vi "BRig_RT__Case_Exp__recordAnalogInput__PortC__fifo__1value__v2.vi"(2 "input_iOccurence":u16, 3 "resetOccurrence":bool, 4 "input_dataCurrent":u16[](array[numeric]), 5 "input_AnaIn_array":i16[][](array[numeric]), 6 "input_iState_start":T1, 7 "rt fifo":refnum<k33>, 8 "input_iState_end":T1, 9 "input_fifo_error":errorcluster) -> (11 "output_fifo_error":errorcluster, 13 "rt fifo out":refnum<k33>, 16 "output_iOccurrence":u16)   [LabVIEW 2014]
uses:
  myRIO_BRig_RT__Case_Exp_stateList.ctl
panel:
  out "anyTimeout":bool
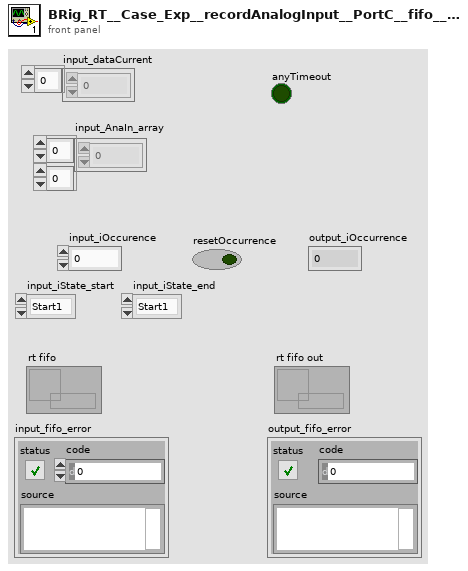
[diagram p1: front panel]
types:
  T1 = typedef "myRIO_BRig_RT__Case_Exp_stateList.ctl" = enum16{"Start1", "Start2", "Start3", "saveSettings1", "saveSettings2", "saveSettings3", "saveSettings4", "saveSettings_LC_ENL_l1", "saveSettings_LC_ENL_l2", "saveSettings_LC_Cue_l1", "saveSettings_LC_Cue_l2", "saveSettings6_LC_l1_Other", "SaveSettings6_LC_l2_Other", "setSettings_Audio", "setSettings_Laser", "initBlock_pre", "initBlock", "initBlock2", "initBlock_post", "initTrial_pre", "initTrial", "initTrial2", "initTrial3", "initTrial4", "initTrial_LC_ENL1", "initTrial_LC_Cue1", "initTrial_LC_Cue1_2", "initTrial_LC_Sel", "initTrial_post", "ENL1_pre", "ENL1", "ENL1_post", "ENL1Penalty_pre", "ENL1Penalty", "ENL2_pre", "ENL2", "ENL2Penalty_pre", "ENL2Penalty", "Cue1_pre", "Cue1", "Cue1_post", "Cue1Penalty_pre", "Cue1Penalty", "Cue2_pre", "Cue2", "Cue2Penalty_pre", "Cue2Penalty", "Selection_pre", "Selection", "Select_post", "SelectReward_pre", "SelectReward", "SelectRewardPost_pre", "SelectRewardPost", "SelectWrong_pre", "SelectWrong", "SelectWrong_post", "SelectTimeout_pre", "SelectTimeout", "SelectTimeout_post", "endTrial_pre", "endTrial1", "endTrial2", "endTrial3", "endTrial_post", "endBlock_pre", "endBlock", "endBlock_post", "endExp", "commConnect", "commUpload_pre", "commUpload_dataBlock", "commUpload_dataCurrent", "commUpload_dataExp", "commUpload_dataLC", "commUpload_dataTrial", "commUpload_post", "saveData_pre", "saveData_dataBlock", "saveData_dataCurrent", "saveData_dataExp", "saveData_dataLC", "saveData_dataTrial", "saveData_post", "empty_endBlock1", "empty_endBlock2", "empty_endTrial1", "empty_endTrial2", "empty_endTrial3", "empty_endTrial4", "empty_endTrial5", "dummyState", "dummyState_endBlock", "FreeReward_pre", "FreeReward", "FreeRewardPost_pre", "FreeRewardPost"}
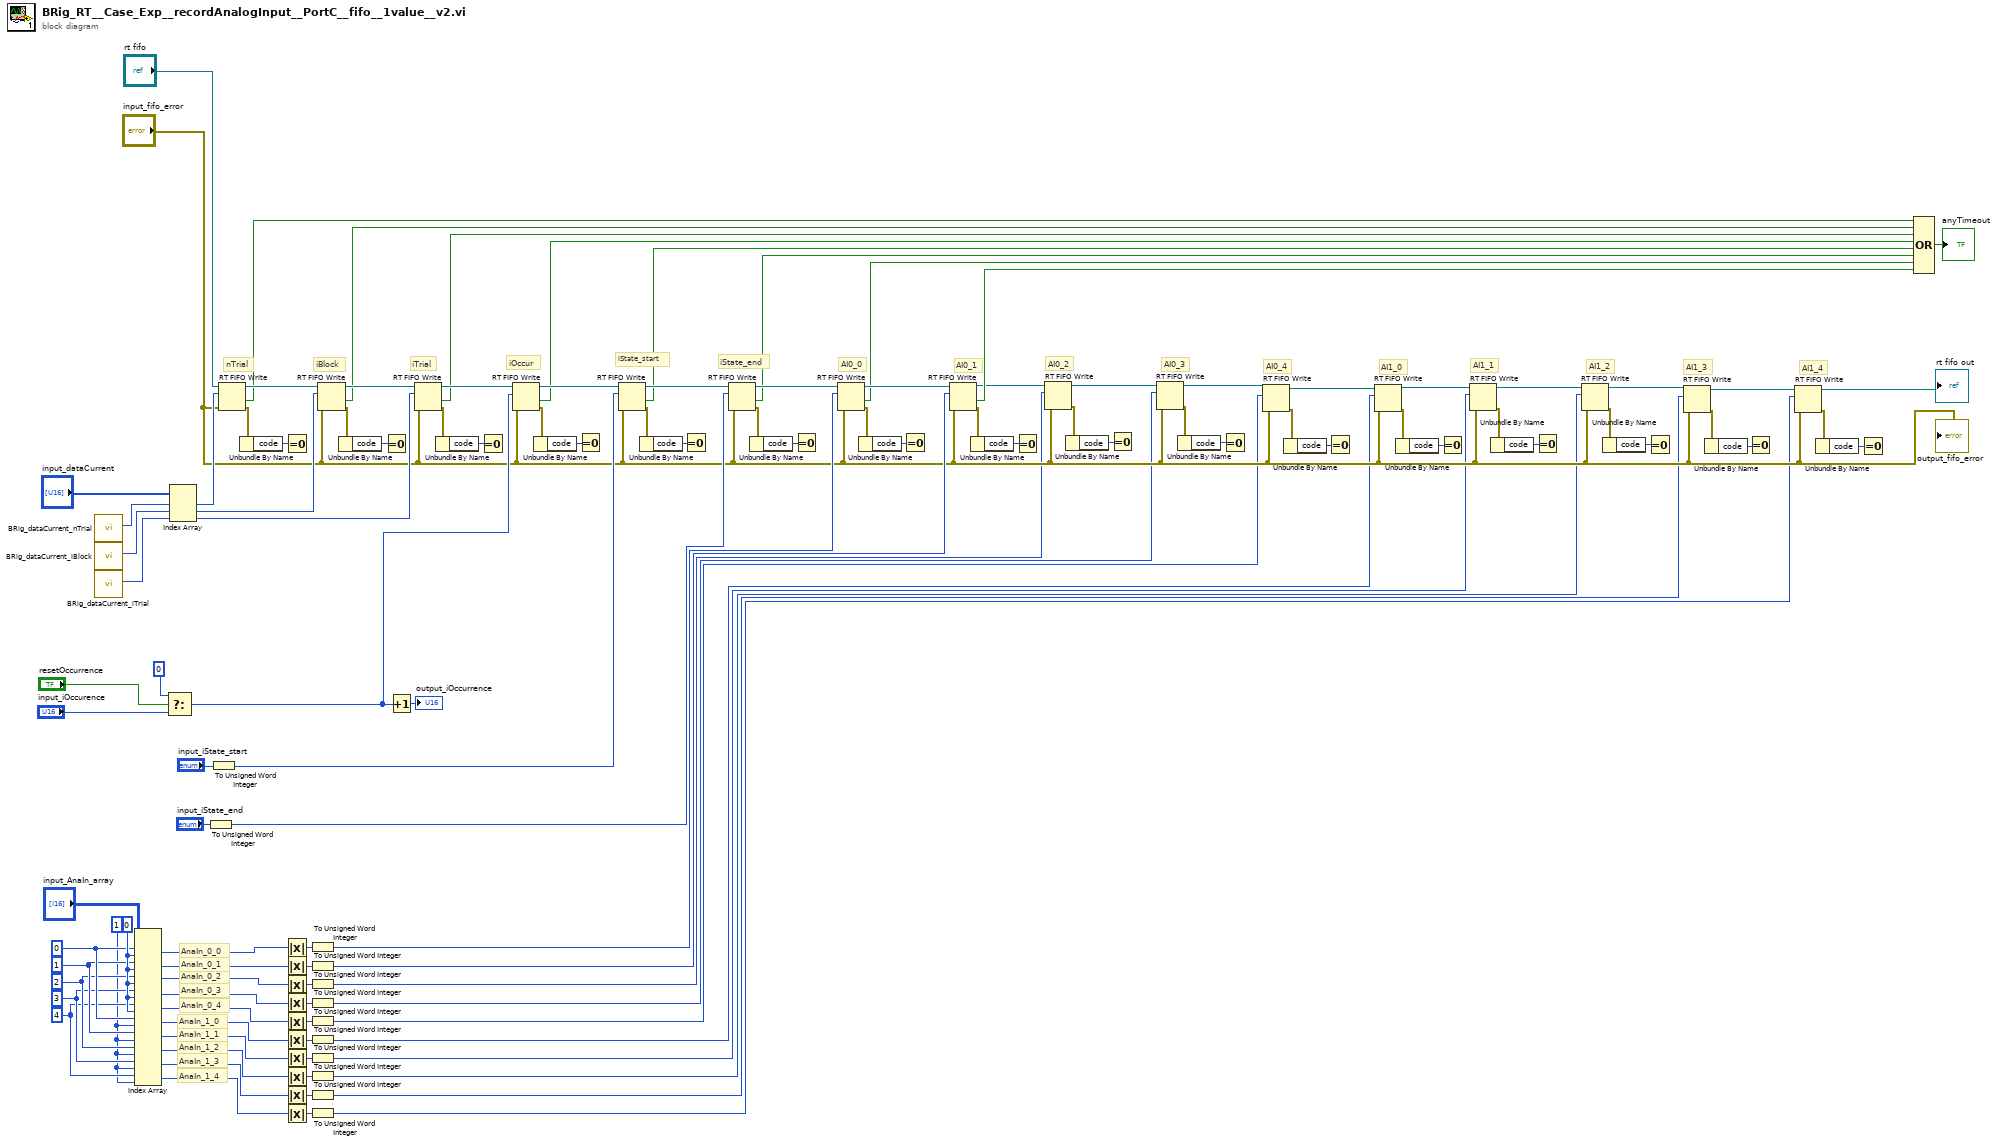
[diagram p0: block diagram]
diagram:
  w53 = 1 ("milliseconds to wait")
  w59 = 0 ("milliseconds to wait")
  w54 = 4 ("milliseconds to wait")
  w55 = 3 ("milliseconds to wait")
  w56 = 2 ("milliseconds to wait")
  w57 = 1 ("milliseconds to wait")
  w58 = 0 ("milliseconds to wait")
  # "AI1_4"
  # "AI1_3"
  # "AI1_2"
  # "AI1_1"
  # "AI1_0"
  # "AI0_4"
  # "AI0_3"
  # "AI0_2"
  # "AnaIn_1_4"
  # "AnaIn_1_3"
  # "AnaIn_1_2"
  # "AnaIn_1_1"
  # "AnaIn_1_0"
  # "AnaIn_0_4"
  # "AnaIn_0_3"
  # "AnaIn_0_2"
  # "AnaIn_0_1"
  # "AnaIn_0_0"
  # "AI0_1"
  # "AI0_0"
  # "iState_end"
  # "iState_start"
  # "iOccur"
  # "iTrial"
  # "iBlock"
  # "nTrial"
  n1 = call "BRig_dataCurrent_nTrial.vi"() -> ("output_nTrial"=w110:i32)  [unwired: 11 in]
  n2 = call "BRig_dataCurrent_iBlock.vi"() -> ("output_iBlock"=w109:i32)  [unwired: 11 in]
  n3 = call "BRig_dataCurrent_iTrial.vi"() -> ("output_iTrial"=w108:i32)  [unwired: 11 in]
  n4 = Index Array(array="input_AnaIn_array", index (row) #1=w58, index (col) #1=w59, index (row) #2=w57, index (col) #2=w59, index (row) #3=w56, index (col) #3=w59, index (row) #4=w55, index (col) #4=w59, index (row) #5=w54, index (col) #5=w59, index (row) #6=w58, index (col) #6=w53, index (row) #7=w57, index (col) #7=w53, index (row) #8=w56, index (col) #8=w53, index (row) #9=w55, index (col) #9=w53, index (row) #10=w54, index (col) #10=w53) -> (element #1=w52:i16, element #2=w51:i16, element #3=w48:i16, element #4=w47:i16, element #5=w42:i16, element #6=w41:i16, element #7=w40:i16, element #8=w39:i16, element #9=w36:i16, element #10=w35:i16)
  n5 = Select(t=u16 0, s="resetOccurrence", f="input_iOccurence") -> (s? t:f=w74:u16)
  n6 = Index Array(array="input_dataCurrent", index #1=w110, index #2=w109, index #3=w108) -> (element #1=w77:u16, element #2=w76:u16, element #3=w75:u16)
  n7 = To Unsigned Word Integer(number="input_iState_end") -> (unsigned 16bit integer=w72:u16)
  n8 = To Unsigned Word Integer(number="input_iState_start") -> (unsigned 16bit integer=w73:u16)
  n9 = RT FIFO Write(0:"rt fifo", 1:w77, 3:"input_fifo_error") -> (8:w95:refnum<k33>, 10:w62:bool, 11:w94:errorcluster)  [unwired: 2 in, 1 out]
  n10 = Unbundle By Name(w94) -> ("code"=w99:i32)
  n11 = Equal To 0?(x=w99) -> ()  [unwired: 1 out]
  n12 = Absolute Value(x=w52) -> (abs(x)=w113:i16)
  n13 = Absolute Value(x=w51) -> (abs(x)=w112:i16)
  n14 = Absolute Value(x=w48) -> (abs(x)=w50:i16)
  n15 = Absolute Value(x=w47) -> (abs(x)=w49:i16)
  n16 = Absolute Value(x=w42) -> (abs(x)=w46:i16)
  n17 = Absolute Value(x=w41) -> (abs(x)=w45:i16)
  n18 = Absolute Value(x=w40) -> (abs(x)=w44:i16)
  n19 = Absolute Value(x=w39) -> (abs(x)=w43:i16)
  n20 = Absolute Value(x=w36) -> (abs(x)=w38:i16)
  n21 = Absolute Value(x=w35) -> (abs(x)=w37:i16)
  n22 = To Unsigned Word Integer(number=w113) -> (unsigned 16bit integer=w71:u16)
  n23 = To Unsigned Word Integer(number=w112) -> (unsigned 16bit integer=w70:u16)
  n24 = To Unsigned Word Integer(number=w50) -> (unsigned 16bit integer=w9:u16)
  n25 = To Unsigned Word Integer(number=w49) -> (unsigned 16bit integer=w8:u16)
  n26 = To Unsigned Word Integer(number=w46) -> (unsigned 16bit integer=w7:u16)
  n27 = To Unsigned Word Integer(number=w45) -> (unsigned 16bit integer=w6:u16)
  n28 = To Unsigned Word Integer(number=w44) -> (unsigned 16bit integer=w5:u16)
  n29 = To Unsigned Word Integer(number=w43) -> (unsigned 16bit integer=w4:u16)
  n30 = To Unsigned Word Integer(number=w38) -> (unsigned 16bit integer=w3:u16)
  n31 = To Unsigned Word Integer(number=w37) -> (unsigned 16bit integer=w2:u16)
  n32 = RT FIFO Write(0:w95, 1:w76, 3:"input_fifo_error") -> (8:w91:refnum<k33>, 10:w63:bool, 11:w97:errorcluster)  [unwired: 2 in, 1 out]
  n33 = Unbundle By Name(w97) -> ("code"=w96:i32)
  n34 = Equal To 0?(x=w96) -> ()  [unwired: 1 out]
  n35 = Increment(x=w74) -> (x+1=→"output_iOccurrence":u16)
  n36 = RT FIFO Write(0:w91, 1:w75, 3:"input_fifo_error") -> (8:w88:refnum<k33>, 10:w64:bool, 11:w93:errorcluster)  [unwired: 2 in, 1 out]
  n37 = Unbundle By Name(w93) -> ("code"=w92:i32)
  n38 = Equal To 0?(x=w92) -> ()  [unwired: 1 out]
  n39 = RT FIFO Write(0:w88, 1:w74, 3:"input_fifo_error") -> (8:w85:refnum<k33>, 10:w65:bool, 11:w89:errorcluster)  [unwired: 2 in, 1 out]
  n40 = Unbundle By Name(w89) -> ("code"=w90:i32)
  n41 = Equal To 0?(x=w90) -> ()  [unwired: 1 out]
  n42 = RT FIFO Write(0:w85, 1:w73, 3:"input_fifo_error") -> (8:w82:refnum<k33>, 10:w66:bool, 11:w86:errorcluster)  [unwired: 2 in, 1 out]
  n43 = Unbundle By Name(w86) -> ("code"=w87:i32)
  n44 = Equal To 0?(x=w87) -> ()  [unwired: 1 out]
  n45 = RT FIFO Write(0:w82, 1:w72, 3:"input_fifo_error") -> (8:w79:refnum<k33>, 10:w67:bool, 11:w83:errorcluster)  [unwired: 2 in, 1 out]
  n46 = Unbundle By Name(w83) -> ("code"=w84:i32)
  n47 = Equal To 0?(x=w84) -> ()  [unwired: 1 out]
  n48 = RT FIFO Write(0:w79, 1:w71, 3:"input_fifo_error") -> (8:w78:refnum<k33>, 10:w68:bool, 11:w80:errorcluster)  [unwired: 2 in, 1 out]
  n49 = Unbundle By Name(w80) -> ("code"=w81:i32)
  n50 = Equal To 0?(x=w81) -> ()  [unwired: 1 out]
  n51 = RT FIFO Write(0:w78, 1:w70, 3:"input_fifo_error") -> (8:w29:refnum<k33>, 10:w69:bool, 11:w100:errorcluster)  [unwired: 2 in, 1 out]
  n52 = Unbundle By Name(w100) -> ("code"=w101:i32)
  n53 = Equal To 0?(x=w101) -> ()  [unwired: 1 out]
  n54 = RT FIFO Write(0:w29, 1:w9, 3:"input_fifo_error") -> (8:w30:refnum<k33>, 11:w31:errorcluster)  [unwired: 2 in, 2 out]
  n55 = Unbundle By Name(w31) -> ("code"=w32:i32)
  n56 = Equal To 0?(x=w32) -> ()  [unwired: 1 out]
  n57 = RT FIFO Write(0:w30, 1:w8, 3:"input_fifo_error") -> (8:w17:refnum<k33>, 11:w33:errorcluster)  [unwired: 2 in, 2 out]
  n58 = Unbundle By Name(w33) -> ("code"=w34:i32)
  n59 = Equal To 0?(x=w34) -> ()  [unwired: 1 out]
  n60 = RT FIFO Write(0:w17, 1:w7, 3:"input_fifo_error") -> (8:w24:refnum<k33>, 11:w25:errorcluster)  [unwired: 2 in, 2 out]
  n61 = Unbundle By Name(w25) -> ("code"=w26:i32)
  n62 = Equal To 0?(x=w26) -> ()  [unwired: 1 out]
  n63 = RT FIFO Write(0:w24, 1:w6, 3:"input_fifo_error") -> (8:w18:refnum<k33>, 11:w27:errorcluster)  [unwired: 2 in, 2 out]
  n64 = Unbundle By Name(w27) -> ("code"=w28:i32)
  n65 = Equal To 0?(x=w28) -> ()  [unwired: 1 out]
  n66 = RT FIFO Write(0:w18, 1:w5, 3:"input_fifo_error") -> (8:w19:refnum<k33>, 11:w20:errorcluster)  [unwired: 2 in, 2 out]
  n67 = Unbundle By Name(w20) -> ("code"=w21:i32)
  n68 = Equal To 0?(x=w21) -> ()  [unwired: 1 out]
  n69 = RT FIFO Write(0:w19, 1:w4, 3:"input_fifo_error") -> (8:w11:refnum<k33>, 11:w22:errorcluster)  [unwired: 2 in, 2 out]
  n70 = Unbundle By Name(w22) -> ("code"=w23:i32)
  n71 = Equal To 0?(x=w23) -> ()  [unwired: 1 out]
  n72 = RT FIFO Write(0:w11, 1:w3, 3:"input_fifo_error") -> (8:w12:refnum<k33>, 11:w13:errorcluster)  [unwired: 2 in, 2 out]
  n73 = Unbundle By Name(w13) -> ("code"=w14:i32)
  n74 = Equal To 0?(x=w14) -> ()  [unwired: 1 out]
  n75 = RT FIFO Write(0:w12, 1:w2, 3:"input_fifo_error") -> (8:→"rt fifo out":refnum<k33>, 11:w15:errorcluster)  [unwired: 2 in, 2 out]
  n76 = Unbundle By Name(w15) -> ("code"=w16:i32)
  n77 = Equal To 0?(x=w16) -> ()  [unwired: 1 out]
  n78 = Compound Arithmetic op=OR(w62, w63, w64, w65, w66, w67, w68, w69) -> (→"anyTimeout":bool)
  "output_fifo_error" <- "input_fifo_error"
